vi "2048.vi"() -> ()   [LabVIEW 2018]
panel:
  in  "Game Over":string="Game Over"
  in  "Winner":string="Winner"
  in  "Colors":u32[](array[colorbox])=[12369084, 13881005, 10130036, 16761177, 16736768, 11814144, 14419712, 13469951, 4991743, 4376575, 8978358, 3126272]
  out "Tiles":refnum<vi>[][](array[refnum])
  in  "Tile 16":bool
  in  "Tile 15":bool
  in  "Tile 14":bool
  in  "Tile 13":bool
  in  "Tile 12":bool
  in  "Tile 11":bool
  in  "Tile 10":bool
  in  "Tile 9":bool
  in  "Tile 8":bool
  in  "Tile 7":bool
  in  "Tile 6":bool
  in  "Tile 5":bool
  in  "Tile 4":bool
  in  "Tile 3":bool
  in  "Tile 2":bool
  in  "Tile 1":bool
  in  "New Game":bool
  out "Score":dbl
  in  "Exit":bool
  in  "Down":bool
  in  "Up":bool
  in  "Right":bool
  in  "Left":bool
  in  "Board":i32[][](array[numeric])=[[0, 0, 0, 0], [0, 0, 0, 0], [0, 0, 0, 0], [0, 0, 0, 0]]
  # "Overview: This example is a LabVIEW version of the number game 2048.\nRequirements: LabVIEW 2012 (or compatible)\nInstructions:\n1.Run the VI\n2.Use the the left, right, up, and down arrows to slide number"
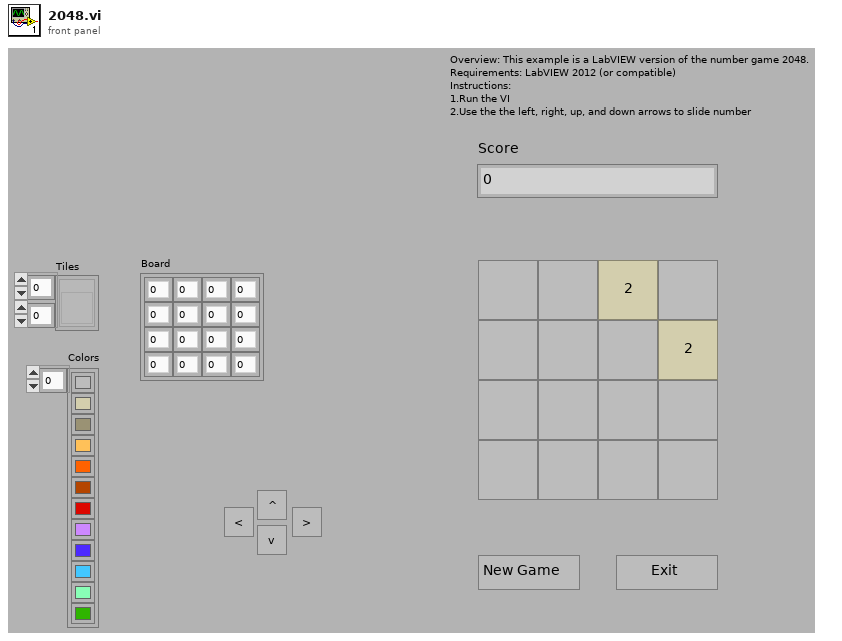
[diagram p1: front panel]
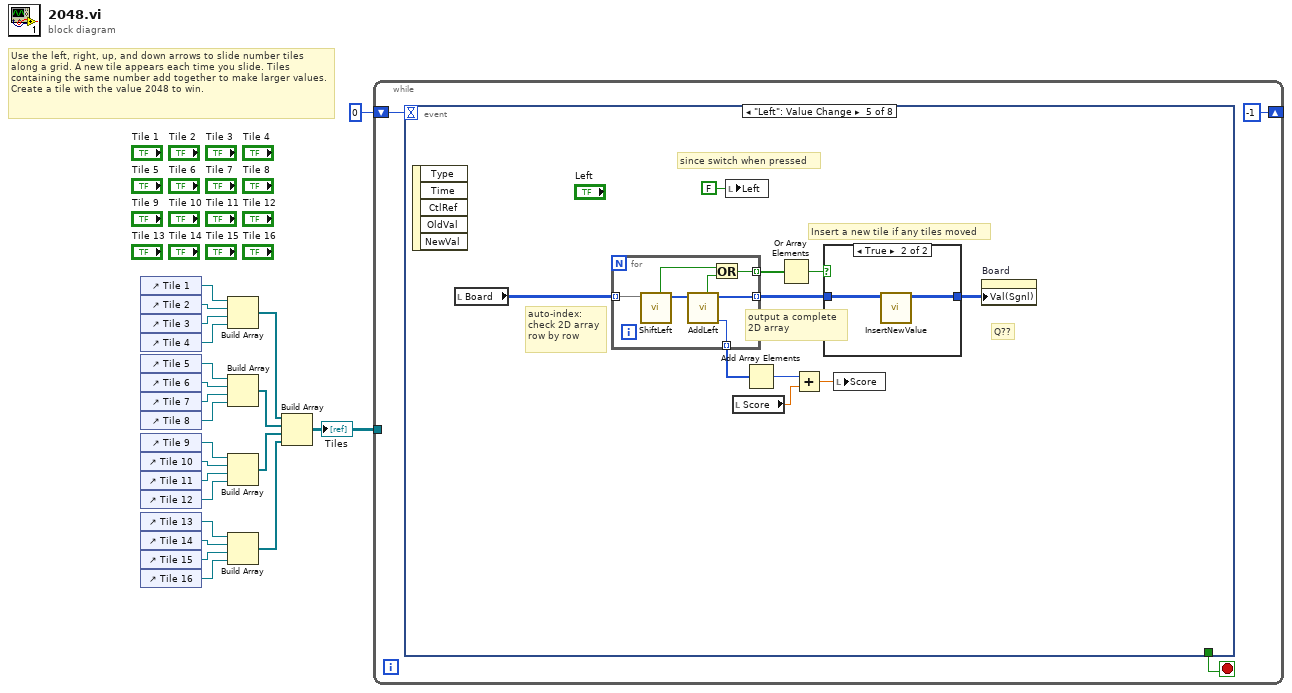
[diagram p0: block diagram]
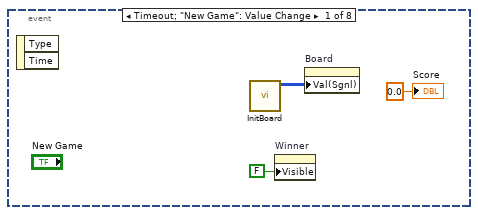
[diagram p2: hidden frame]
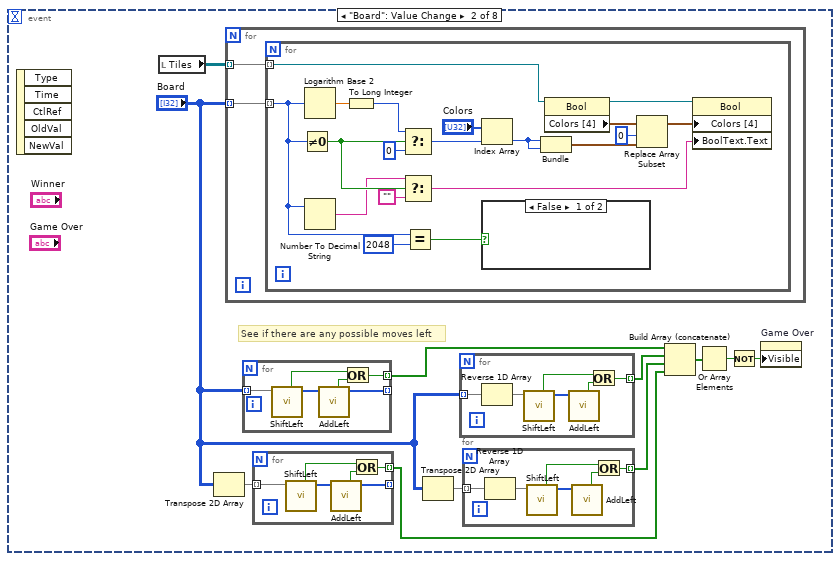
[diagram p3: hidden frame]
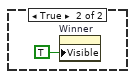
[diagram p4: hidden frame]
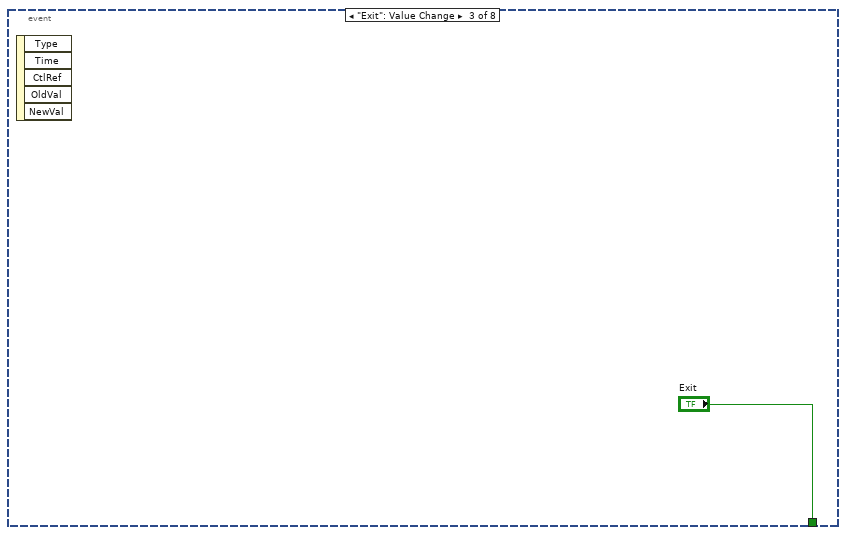
[diagram p5: hidden frame]
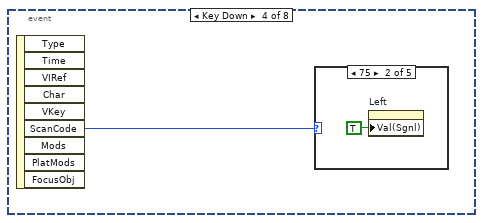
[diagram p6: hidden frame]
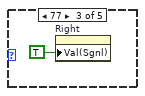
[diagram p8: hidden frame]
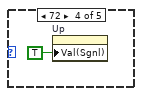
[diagram p9: hidden frame]
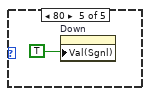
[diagram p10: hidden frame]
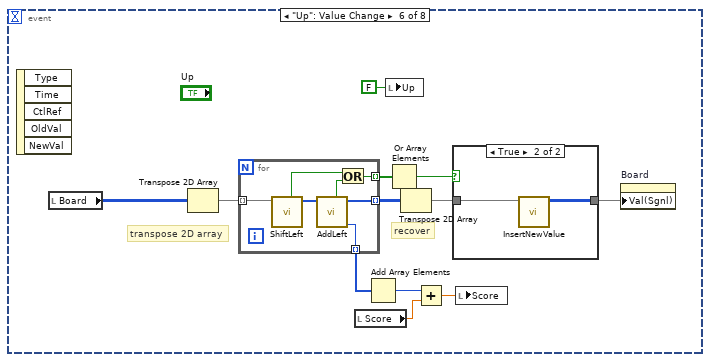
[diagram p12: hidden frame]
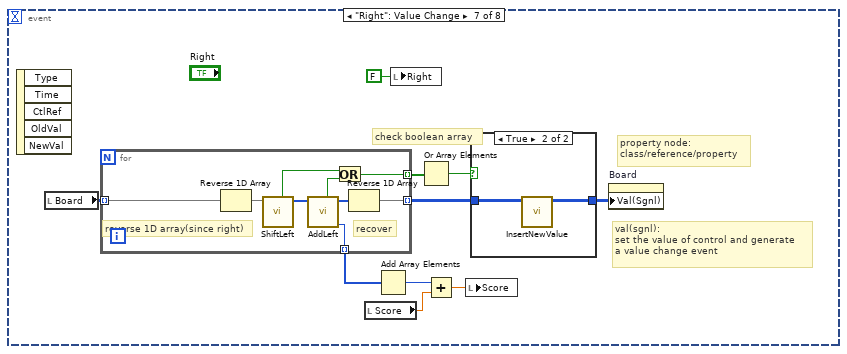
[diagram p14: hidden frame]
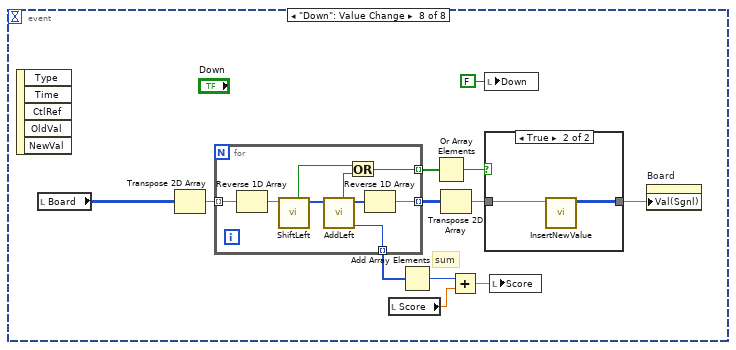
[diagram p16: hidden frame]
diagram:
  # "Use the left, right, up, and down arrows to slide number tiles along a grid. A new tile appears each time you slide. Tiles containing the same number add together to make larger values. Create a tile with the value 2048 to win."
  n1 = control-ref of="Tile 1"() -> (w21:refnum<vi>)
  n2 = control-ref of="Tile 2"() -> (w20:refnum<vi>)
  n3 = control-ref of="Tile 3"() -> (w19:refnum<vi>)
  n4 = control-ref of="Tile 4"() -> (w18:refnum<vi>)
  n5 = control-ref of="Tile 5"() -> (w14:refnum<vi>)
  n6 = control-ref of="Tile 6"() -> (w15:refnum<vi>)
  n7 = control-ref of="Tile 7"() -> (w16:refnum<vi>)
  n8 = control-ref of="Tile 8"() -> (w17:refnum<vi>)
  n9 = control-ref of="Tile 9"() -> (w13:refnum<vi>)
  n10 = control-ref of="Tile 10"() -> (w12:refnum<vi>)
  n11 = control-ref of="Tile 11"() -> (w11:refnum<vi>)
  n12 = control-ref of="Tile 12"() -> (w10:refnum<vi>)
  n13 = control-ref of="Tile 13"() -> (w6:refnum<vi>)
  n14 = control-ref of="Tile 14"() -> (w7:refnum<vi>)
  n15 = control-ref of="Tile 15"() -> (w8:refnum<vi>)
  n16 = control-ref of="Tile 16"() -> (w9:refnum<vi>)
  n17 = Build Array(w21, w20, w19, w18) -> (w5:refnum<vi>[])
  n18 = Build Array(w14, w15, w16, w17) -> (w3:refnum<vi>[])
  n19 = Build Array(w13, w12, w11, w10) -> (w2:refnum<vi>[])
  n20 = Build Array(w6, w7, w8, w9) -> (w4:refnum<vi>[])
  n21 = Build Array(w5, w3, w2, w4) -> (w1:refnum<vi>[][])
  "Tiles" <- w1
  n22 = while {
    shift-right: [-1] -> _
    shift-left: 0 -> [w23]
    tunnel: w1 -> [_]
    stop <- w25 stop-if-true
    n23 = event shown="[4] \"Left\": Value Change" {
      selector: _ -> [_ _ _ _ _ _ _ _]
      dyn-events: _ -> [_ _ _ _ _ _ _ _]
      timeout: w23 -> [_ _ _ _ _ _ _ _]
      tunnel: [_ _ "Exit" _ _ _ _ _] -> w25
      event Timeout; "New Game": Value Change {
        n24 = event-data() -> ()  [unwired: 1 in, 2 out]
        n25 = call "InitBoard.vi"() -> ("output array"=w27:i32[][])  [unwired: 11 in]
        n26 = property on="Winner" class="Str"("Visible"=FALSE) -> ()  [unwired: 2 in, 2 out]
        n27 = property on="Board" class="Arr (strict)"("Val(Sgnl)"=w27) -> ()  [unwired: 2 in, 2 out]
        "Score" <- 0.0 ("score")
      }
      event "Board": Value Change {
        # "See if there are any possible moves left"
        n28 = event-data() -> ()  [unwired: 1 in, 5 out]
        n29 = local read "Tiles"() -> (w39:refnum<vi>[][])
        n30 = Transpose 2D Array(2D array="Board") -> (transposed array=w38:i32[][])
        n31 = for {
          tunnel: "Board" -> [w64] mode=indexing
          tunnel: w39 -> [w65] mode=indexing
          n32 = for {
            tunnel: w65 -> [w70] mode=indexing
            tunnel: w64 -> [w68] mode=indexing
            n33 = Not Equal To 0?(x=w68) -> (x != 0?=w76:bool)
            n34 = Logarithm Base 2(1:w68) -> (0:w81:dbl)
            n35 = Number To Decimal String(number=w68) -> (decimal integer string=w75:string)  [unwired: 1 in]
            n36 = To Long Integer(number=w81) -> (32bit integer=w78:i32)
            n37 = Select(t=w78, s=w76, f=0 ("t")) -> (s? t:f=w80:i32)
            n38 = Select(t=w75, s=w76, f="") -> (s? t:f=w71:string)
            n39 = Equal?(x=w68, y=2048) -> (x = y?=w66:bool)
            n40 = Index Array(array="Colors", index=w80) -> (element=w79:u32)
            n41 = case shown="False" w66 {
              frame False {
              }
              frame True {
                n42 = property on="Winner" class="Str"("Visible"=TRUE) -> ()  [unwired: 2 in, 2 out]
              }
            }
            n43 = Bundle("Color Box 2"=w79, "Color Box 2"=w79) -> (w82:cluster{"Color Box 2":u32, "Color Box 2":u32})  [unwired: 1 in]
            n44 = property on="Property Node" class="Bool"(reference=w70) -> (reference out=w69:refnum<vi>, "Colors [4]"=w84:cluster{u32, u32}[])  [unwired: 1 in, 1 out]
            n45 = Replace Array Subset(array=w84, new element=w82, index=0) -> (w72:cluster{u32, u32}[])
            n46 = property on="Property Node" class="Bool"(reference=w69, "Colors [4]"=w72, "BoolText.Text"=w71) -> ()  [unwired: 1 in, 2 out]
          }
        }
        n47 = for {
          tunnel: "Board" -> [w63] mode=indexing
          tunnel: [w61] -> _ mode=indexing
          tunnel: [w58] -> w35 mode=indexing
          n48 = call "ShiftLeft.vi"("Array"=w63) -> ("Array 2"=w62:i32[], "tiles moved?"=w59:bool)  [unwired: 9 in]
          n49 = call "AddLeft.vi"("Array"=w62) -> ("Array 2"=w61:i32[], "tiles moved?"=w60:bool)  [unwired: 8 in, 1 out]
          n50 = Or(x=w59, y=w60) -> (x .or. y?=w58:bool)
        }
        n51 = for {
          tunnel: w38 -> [w57] mode=indexing
          tunnel: [w55] -> _ mode=indexing
          tunnel: [w52] -> w33 mode=indexing
          n52 = call "ShiftLeft.vi"("Array"=w57) -> ("Array 2"=w56:i32[], "tiles moved?"=w53:bool)  [unwired: 9 in]
          n53 = call "AddLeft.vi"("Array"=w56) -> ("Array 2"=w55:i32[], "tiles moved?"=w54:bool)  [unwired: 8 in, 1 out]
          n54 = Or(x=w53, y=w54) -> (x .or. y?=w52:bool)
        }
        n55 = Transpose 2D Array(2D array="Board") -> (transposed array=w37:i32[][])
        n56 = for {
          tunnel: "Board" -> [w50] mode=indexing
          tunnel: [w46] -> w34 mode=indexing
          n57 = Reverse 1D Array(array=w50) -> (reversed array=w49:i32[])
          n58 = call "ShiftLeft.vi"("Array"=w49) -> ("Array 2"=w51:i32[], "tiles moved?"=w47:bool)  [unwired: 9 in]
          n59 = call "AddLeft.vi"("Array"=w51) -> ("tiles moved?"=w48:bool)  [unwired: 8 in, 2 out]
          n60 = Or(x=w47, y=w48) -> (x .or. y?=w46:bool)
        }
        n61 = for {
          tunnel: w37 -> [w44] mode=indexing
          tunnel: [w40] -> w32 mode=indexing
          n62 = Reverse 1D Array(array=w44) -> (reversed array=w43:i32[])
          n63 = call "ShiftLeft.vi"("Array"=w43) -> ("Array 2"=w45:i32[], "tiles moved?"=w41:bool)  [unwired: 9 in]
          n64 = call "AddLeft.vi"("Array"=w45) -> ("tiles moved?"=w42:bool)  [unwired: 8 in, 2 out]
          n65 = Or(x=w41, y=w42) -> (x .or. y?=w40:bool)
        }
        n66 = Build Array (concatenate)(w35, w34, w32, w33) -> (w31:bool[])
        n67 = Or Array Elements(Boolean array=w31) -> (logical OR=w30:bool)
        n68 = Not(x=w30) -> (.not. x?=w29:bool)
        n69 = property on="Game Over" class="Str"("Visible"=w29) -> ()  [unwired: 2 in, 2 out]
      }
      event "Exit": Value Change {
        n70 = event-data() -> ()  [unwired: 1 in, 5 out]
      }
      event Key Down {
        n71 = event-data() -> ("ScanCode"=w87:i16)  [unwired: 1 in, 8 out]
        n72 = case shown="75" w87 {
          frame 0, Default {
          }
          frame 75 {
            n73 = property on="Left" class="Bool (strict)"("Val(Sgnl)"=TRUE) -> ()  [unwired: 2 in, 2 out]
          }
          frame 77 {
            n74 = property on="Right" class="Bool (strict)"("Val(Sgnl)"=TRUE) -> ()  [unwired: 2 in, 2 out]
          }
          frame 72 {
            n75 = property on="Up" class="Bool (strict)"("Val(Sgnl)"=TRUE) -> ()  [unwired: 2 in, 2 out]
          }
          frame 80 {
            n76 = property on="Down" class="Bool (strict)"("Val(Sgnl)"=TRUE) -> ()  [unwired: 2 in, 2 out]
          }
        }
      }
      event "Left": Value Change {
        # "output a complete\n2D array"
        # "auto-index:\ncheck 2D array\nrow by row"
        # "since switch when pressed"
        # "Q??"
        # "Insert a new tile if any tiles moved"
        n77 = event-data() -> ()  [unwired: 1 in, 5 out]
        n78 = local read "Board"() -> (w100:i32[][])
        n79 = for {
          tunnel: w100 -> [w111] mode=indexing
          tunnel: [w109] -> w99 mode=indexing
          tunnel: [w108] -> w95 mode=indexing
          tunnel: [w105] -> w93 mode=indexing
          n80 = call "ShiftLeft.vi"("Array"=w111) -> ("Array 2"=w110:i32[], "tiles moved?"=w106:bool)  [unwired: 9 in]
          n81 = call "AddLeft.vi"("Array"=w110) -> ("score"=w108:i32, "Array 2"=w109:i32[], "tiles moved?"=w107:bool)  [unwired: 8 in]
          n82 = Or(x=w106, y=w107) -> (x .or. y?=w105:bool)
        }
        n83 = local write "Left"(FALSE ("Left")) -> ()
        n84 = local read "Score"() -> (w96:dbl)
        n85 = Add Array Elements(numeric array=w95) -> (sum=w98:i32)
        n86 = Or Array Elements(Boolean array=w93) -> (logical OR=w92:bool)
        n87 = Add(x=w98, y=w96) -> (x+y=w97:dbl)
        n88 = case shown="True" w92 {
          tunnel: w99 -> [w102 w104]
          tunnel: [w102 w103] -> w94
          frame False {
          }
          frame True {
            n89 = call "InsertNewValue.vi"("Board"=w104) -> ("output"=w103:i32[][])  [unwired: 10 in]
          }
        }
        n90 = local write "Score"(w97) -> ()
        n91 = property on="Board" class="Arr (strict)"("Val(Sgnl)"=w94) -> ()  [unwired: 2 in, 2 out]
      }
      event "Up": Value Change {
        # "recover"
        # "transpose 2D array"
        n92 = event-data() -> ()  [unwired: 1 in, 5 out]
        n93 = local read "Board"() -> (w122:i32[][])
        n94 = Transpose 2D Array(2D array=w122) -> (transposed array=w120:i32[][])
        n95 = for {
          tunnel: w120 -> [w133] mode=indexing
          tunnel: [w131] -> w121 mode=indexing
          tunnel: [w130] -> w115 mode=indexing
          tunnel: [w127] -> w113 mode=indexing
          n96 = call "ShiftLeft.vi"("Array"=w133) -> ("Array 2"=w132:i32[], "tiles moved?"=w128:bool)  [unwired: 9 in]
          n97 = call "AddLeft.vi"("Array"=w132) -> ("score"=w130:i32, "Array 2"=w131:i32[], "tiles moved?"=w129:bool)  [unwired: 8 in]
          n98 = Or(x=w128, y=w129) -> (x .or. y?=w127:bool)
        }
        n99 = local read "Score"() -> (w116:dbl)
        n100 = Add Array Elements(numeric array=w115) -> (sum=w118:i32)
        n101 = local write "Up"(FALSE ("Up")) -> ()
        n102 = Or Array Elements(Boolean array=w113) -> (logical OR=w112:bool)
        n103 = Transpose 2D Array(2D array=w121) -> (transposed array=w119:i32[][])
        n104 = Add(x=w118, y=w116) -> (x+y=w117:dbl)
        n105 = case shown="True" w112 {
          tunnel: w119 -> [w124 w126]
          tunnel: [w124 w125] -> w114
          frame False {
          }
          frame True {
            n106 = call "InsertNewValue.vi"("Board"=w126) -> ("output"=w125:i32[][])  [unwired: 10 in]
          }
        }
        n107 = local write "Score"(w117) -> ()
        n108 = property on="Board" class="Arr (strict)"("Val(Sgnl)"=w114) -> ()  [unwired: 2 in, 2 out]
      }
      event "Right": Value Change {
        # "check boolean array"
        # "property node:\nclass/reference/property"
        # "val(sgnl):\nset the value of control and generate \na value change event"
        n109 = event-data() -> ()  [unwired: 1 in, 5 out]
        n110 = local read "Board"() -> (w142:i32[][])
        n111 = for {
          tunnel: w142 -> [w153] mode=indexing
          tunnel: [w151] -> w141 mode=indexing
          tunnel: [w150] -> w137 mode=indexing
          tunnel: [w147] -> w135 mode=indexing
          # "reverse 1D array(since right)"
          # "recover"
          n112 = Reverse 1D Array(array=w153) -> (reversed array=w152:i32[])
          n113 = call "ShiftLeft.vi"("Array"=w152) -> ("Array 2"=w155:i32[], "tiles moved?"=w148:bool)  [unwired: 9 in]
          n114 = call "AddLeft.vi"("Array"=w155) -> ("score"=w150:i32, "Array 2"=w154:i32[], "tiles moved?"=w149:bool)  [unwired: 8 in]
          n115 = Or(x=w148, y=w149) -> (x .or. y?=w147:bool)
          n116 = Reverse 1D Array(array=w154) -> (reversed array=w151:i32[])
        }
        n117 = local read "Score"() -> (w138:dbl)
        n118 = Add Array Elements(numeric array=w137) -> (sum=w140:i32)
        n119 = local write "Right"(FALSE ("Right")) -> ()
        n120 = Or Array Elements(Boolean array=w135) -> (logical OR=w134:bool)
        n121 = Add(x=w140, y=w138) -> (x+y=w139:dbl)
        n122 = local write "Score"(w139) -> ()
        n123 = case shown="True" w134 {
          tunnel: w141 -> [w144 w146]
          tunnel: [w144 w145] -> w136
          frame False {
          }
          frame True {
            n124 = call "InsertNewValue.vi"("Board"=w146) -> ("output"=w145:i32[][])  [unwired: 10 in]
          }
        }
        n125 = property on="Board" class="Arr (strict)"("Val(Sgnl)"=w136) -> ()  [unwired: 2 in, 2 out]
      }
      event "Down": Value Change {
        # "sum"
        n126 = event-data() -> ()  [unwired: 1 in, 5 out]
        n127 = local read "Board"() -> (w166:i32[][])
        n128 = Transpose 2D Array(2D array=w166) -> (transposed array=w164:i32[][])
        n129 = for {
          tunnel: w164 -> [w177] mode=indexing
          tunnel: [w175] -> w165 mode=indexing
          tunnel: [w174] -> w162 mode=indexing
          tunnel: [w171] -> w157 mode=indexing
          n130 = Reverse 1D Array(array=w177) -> (reversed array=w176:i32[])
          n131 = call "ShiftLeft.vi"("Array"=w176) -> ("Array 2"=w179:i32[], "tiles moved?"=w172:bool)  [unwired: 9 in]
          n132 = call "AddLeft.vi"("Array"=w179) -> ("score"=w174:i32, "Array 2"=w178:i32[], "tiles moved?"=w173:bool)  [unwired: 8 in]
          n133 = Or(x=w172, y=w173) -> (x .or. y?=w171:bool)
          n134 = Reverse 1D Array(array=w178) -> (reversed array=w175:i32[])
        }
        n135 = local read "Score"() -> (w159:dbl)
        n136 = Add Array Elements(numeric array=w162) -> (sum=w161:i32)
        n137 = Or Array Elements(Boolean array=w157) -> (logical OR=w156:bool)
        n138 = Transpose 2D Array(2D array=w165) -> (transposed array=w163:i32[][])
        n139 = Add(x=w161, y=w159) -> (x+y=w160:dbl)
        n140 = local write "Down"(FALSE ("Down")) -> ()
        n141 = case shown="True" w156 {
          tunnel: w163 -> [w168 w170]
          tunnel: [w168 w169] -> w158
          frame False {
          }
          frame True {
            n142 = call "InsertNewValue.vi"("Board"=w170) -> ("output"=w169:i32[][])  [unwired: 10 in]
          }
        }
        n143 = local write "Score"(w160) -> ()
        n144 = property on="Board" class="Arr (strict)"("Val(Sgnl)"=w158) -> ()  [unwired: 2 in, 2 out]
      }
    }
  }
